vi "Pneumatics Command Set Tele.vi"(10 "Solenoid Command":T2, 11 "RT FIFO":u64) -> (3 "Cluster Out":T1)   [LabVIEW 2015]
uses:
  Pneumatics Notifier.ctl
  Pneumatics Command.ctl
  Pneumatics Status.ctl
panel:
  in  "Cluster":T1
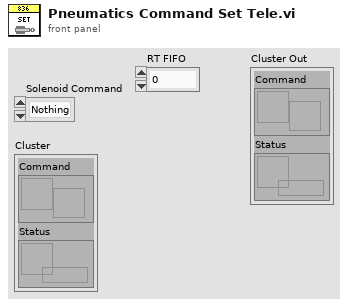
[diagram p1: front panel]
types:
  T1 = typedef "Pneumatics Notifier.ctl" = cluster{"Command":refnum<notifier>, "Status":refnum<queue>}
  T2 = typedef "Pneumatics Command.ctl" = enum16{"Nothing", "Forward", "Reverse", "Toggle"}
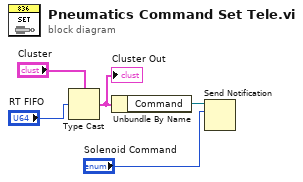
[diagram p0: block diagram]
diagram:
  n1 = Type Cast(type="Cluster", x="RT FIFO") -> (*(type *) &x=w2:T1)
  "Cluster Out" <- w2
  n2 = Unbundle By Name(w2) -> ("Command"=w5:refnum<notifier>)
  n3 = Send Notification(notification="Solenoid Command", notifier=w5) -> ()  [unwired: 1 in, 2 out]
